vi "STFT_PreProcess.vi"(6 "iteration":i32, 9 "FFT info":T1={"FFT block size"=1024, "number of FFT"=0, "start index"=0, "increment"=0.0} {"increment" format="%.2f"}, 11 "Signal in":dbl[](array[numeric])) -> (3 "preprocessed Signal out":dbl[](array[numeric]))   [LabVIEW 2020]
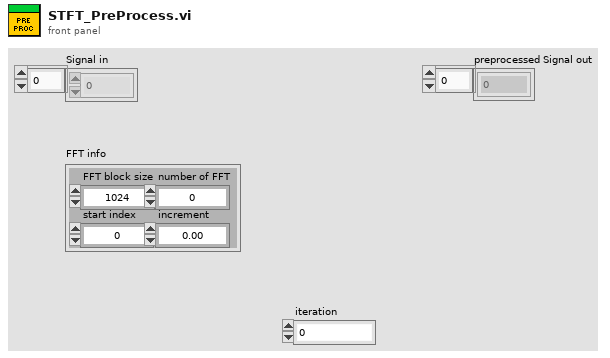
[diagram p1: front panel]
types:
  T1 = cluster{"FFT block size":i32, "number of FFT":i32, "start index":i32, "increment":dbl}
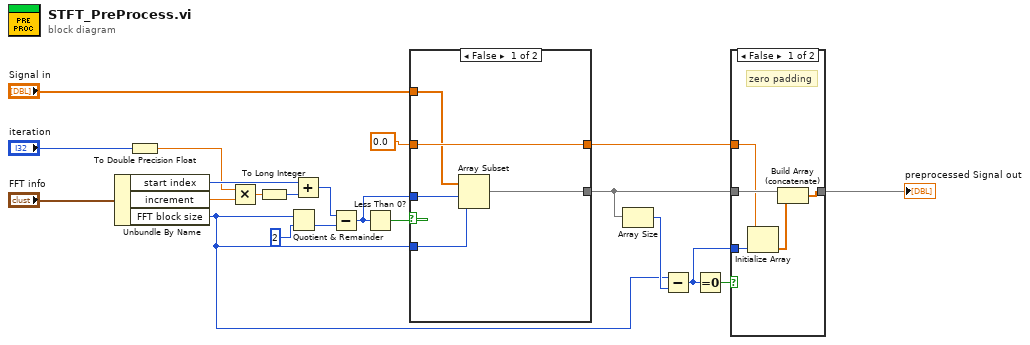
[diagram p0: block diagram]
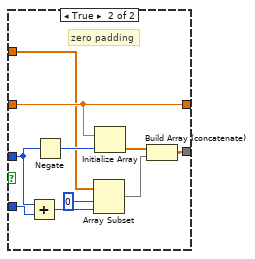
[diagram p2: hidden frame]
diagram:
  n1 = Unbundle By Name("FFT info") -> ("start index"=w8:i32, "increment"=w7:dbl, "FFT block size"=w1:i32)
  n2 = To Double Precision Float(number="iteration") -> (double precision float=w2:dbl)
  n3 = Multiply(x=w2, y=w7) -> (x*y=w10:dbl)
  n4 = To Long Integer(number=w10) -> (32bit integer=w11:i32)
  n5 = Quotient & Remainder(x=w1, y=2) -> (floor(x/y)=w6:i32)  [unwired: 1 out]
  n6 = Add(x=w8, y=w11) -> (x+y=w12:i32)
  n7 = Subtract(x=w12, y=w6) -> (x-y=w5:i32)
  n8 = Less Than 0?(x=w5) -> (x < 0?=w15:bool)
  n9 = case shown="False" w15 {
    tunnel: w1 -> [w25 w30]
    tunnel: [w26 w31] -> w13
    tunnel: w5 -> [w24 w29]
    tunnel: "Signal in" -> [w22 w27]
    tunnel: 0.0 -> [w23 w28]
    tunnel: [w23 w28] -> w3
    frame False {
      n10 = Array Subset(array=w22, index=w24, length=w25) -> (w26:dbl[])
    }
    frame True {
      # "zero padding"
      n11 = Add(x=w29, y=w30) -> (x+y=w34:i32)
      n12 = Negate(x=w29) -> (-x=w36:i32)
      n13 = Array Subset(array=w27, index=0, length=w34) -> (w32:dbl[])
      n14 = Initialize Array(w28, w36) -> (w33:dbl[])
      n15 = Build Array (concatenate)(w33, w32) -> (w31:dbl[])
    }
  }
  n16 = Array Size(array=w13) -> (size(s)=w16:i32)
  n17 = Subtract(x=w1, y=w16) -> (x-y=w14:i32)
  n18 = Equal To 0?(x=w14) -> (x = 0?=w17:bool)
  n19 = case shown="False" w17 {
    tunnel: [w38 w42] -> w19
    tunnel: w13 -> [w41 w42]
    tunnel: w14 -> [w40 _]
    tunnel: w3 -> [w37 _]
    frame False {
      # "zero padding"
      n20 = Initialize Array(w37, w40) -> (w39:dbl[])
      n21 = Build Array (concatenate)(w41, w39) -> (w38:dbl[])
    }
    frame True {
    }
  }
  "preprocessed Signal out" <- w19
